vi "Get Serial Number.vi"(8 "error in":errorcluster, 11 "VISA resource in":refnum<visa-resource-name>) -> (0 "error out":errorcluster, 1 "found?":bool, 2 "serial number":string, 3 "VISA resource out":refnum<visa-resource-name>, 5 "CALSTR":string)   [LabVIEW 2020, in "3458A Virtual Digitizer.lvlib" / "3458A Digitizing Low Levels.lvlib"]
doc: "Reads calibration string from 3458A unit and scans for serial number in it. All possible serial number formats for HP, Agilent and Keysight are considered. The serial number can be inserted anywhere in the calibration string. Examples of supported formats:\n'US12345678', '2823A 12345', '2823A-12345'\n\nNote: Reentrant VI so it can be executed in parallel for multiple 3458A sessions."
uses:
  3458A Digitizing Low Levels/3458A Digitizing Low Levels.lvlib
  <vilib>/regexp/Match Regular Expression.xnode
  3458A Basic Driver.lvlib
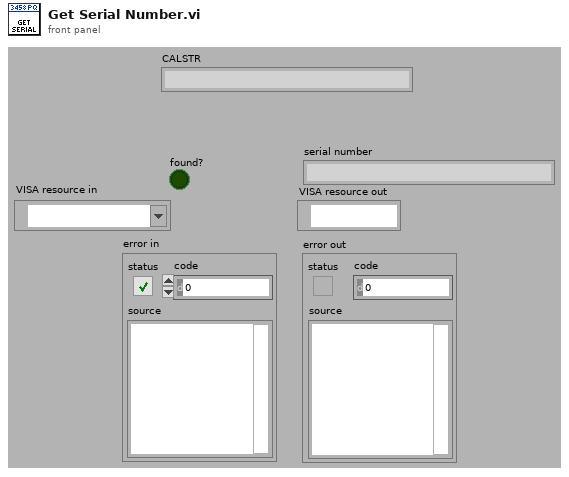
[diagram p1: front panel]
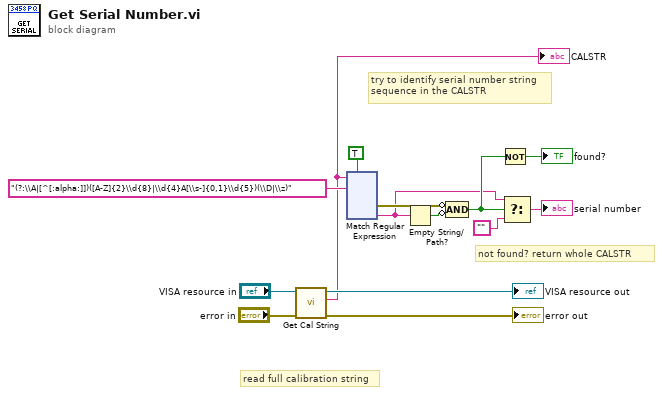
[diagram p0: block diagram]
diagram:
  # "not found? return whole CALSTR"
  # "try to identify serial number string\nsequence in the CALSTR"
  # "read full calibration string"
  n1 = call "Get Cal String.vi"("error in(no error)"="error in", "VISA Resource Name"="VISA resource in") -> ("error out"=→"error out":errorcluster, "calibration string"=w1:string, "VISA resource name out"=→"VISA resource out":refnum<visa-resource-name>)  [unwired: 7 in]
  "CALSTR" <- w1
  n2 = xnode "Match Regular Expression"("input string"=w1, "regular expression"="(?:\\A|[^[:alpha:]])([A-Z]{2}\\d{8}|\\d{4}A[\\s-]{0,1}\\d{5})(\\D|\\z)", "ignore case? (F)"=TRUE) -> ("error out"=w9:errorcluster, "submatch 1"=w3:string)  [unwired: 3 in, 4 out]
  n3 = Empty String/Path?(string/path=w3) -> (empty?=w8:bool)
  n4 = Compound Arithmetic op=AND(invert w9, invert w8) -> (w7:bool)
  n5 = Not(x=w7) -> (.not. x?=→"found?":bool)
  n6 = Select(t=w3, s=w7, f="") -> (s? t:f=→"serial number":string)
